vi "校准测试.vi"(8 "error in (no error)":errorcluster, 9 "out":i32=1, 11 "in":i32=2) -> (0 "error out":errorcluster)   [LabVIEW 2015]
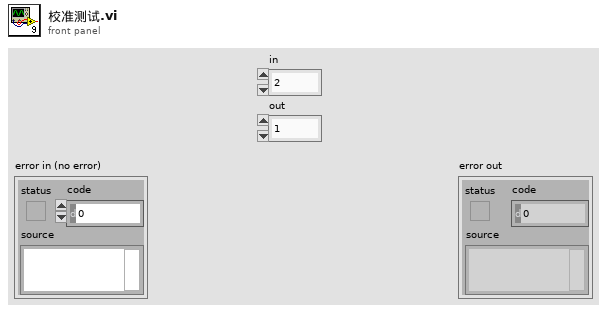
[diagram p1: front panel]
types:
  T1 = typedef "直通基准state.ctl" = enum16{"Idle", "开始消息", "切换开关", "网分测量", "数据库操作", "结束消息"}
  T2 = cluster{"Freq":dbl[], "S11":dbl[], "S12":dbl[], "S21":dbl[], "S22":dbl[]}
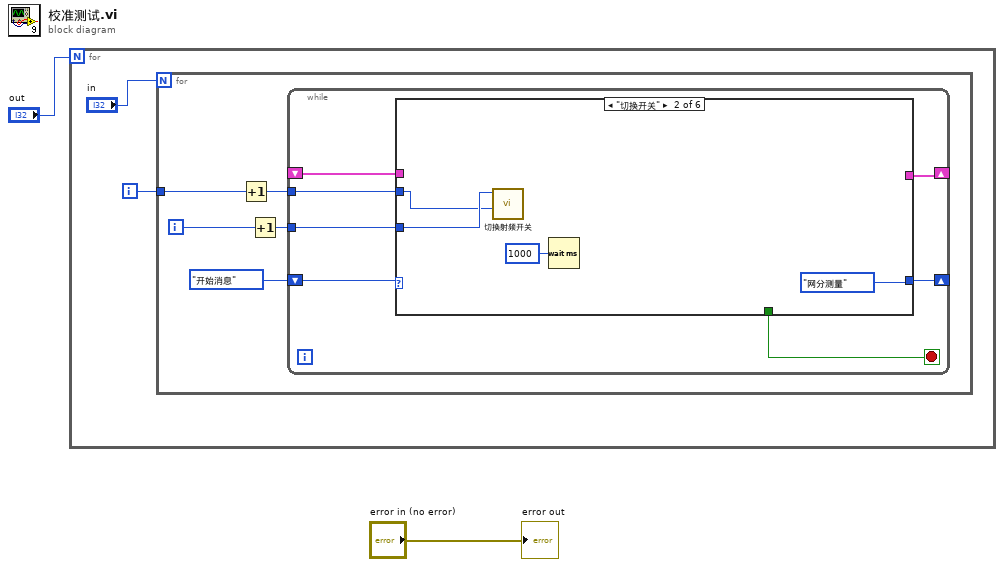
[diagram p0: block diagram]
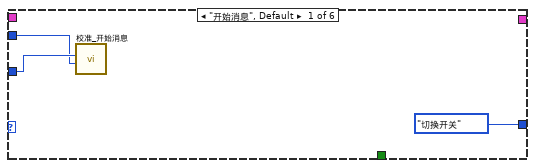
[diagram p2: hidden frame]
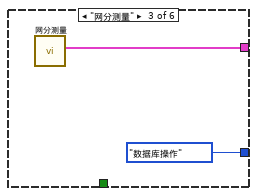
[diagram p3: hidden frame]
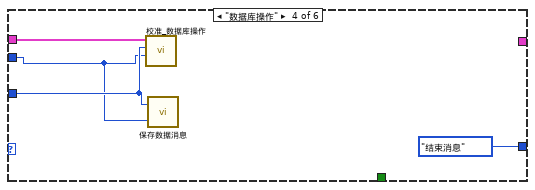
[diagram p4: hidden frame]
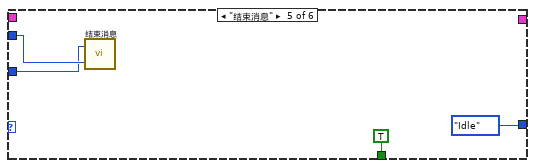
[diagram p5: hidden frame]
diagram:
  n1 = for {
    N: "out" -> [_]
    i -> [w4]
    n2 = for {
      N: "in" -> [_]
      tunnel: w4 -> [w9]
      i -> [w8]
      n3 = Increment(x=w9) -> (x+1=w7:i32)
      n4 = Increment(x=w8) -> (x+1=w6:i32)
      n5 = while {
        tunnel: w7 -> [w16]
        tunnel: w6 -> [w15]
        shift-right: [w13] -> _
        shift-left: 直通基准state."开始消息" ("直通基准State") -> [w14]
        shift-right: [w11] -> _
        shift-left: _ -> [w10]
        stop <- w12 stop-if-true
        n6 = case shown="\"切换开关\"" w14 {
          tunnel: w16 -> [w17 w20 _ w26 w31 _]
          tunnel: w15 -> [w18 w21 _ w27 w30 _]
          tunnel: [直通基准state."切换开关" ("直通基准State") 直通基准state."网分测量" ("直通基准State") 直通基准state."数据库操作" ("直通基准State") 直通基准state."结束消息" ("直通基准State") 直通基准state."Idle" ("直通基准State") _] -> w13
          tunnel: [_ _ _ _ TRUE _] -> w12
          tunnel: [_ _ w25 _ _ _] -> w11
          tunnel: w10 -> [_ _ _ w29 _ _]
          frame "开始消息", Default {
            n7 = call "校准_开始消息.vi"("COM"=w17, "A"=w18) -> ()  [unwired: 10 in]
          }
          frame "切换开关" {
            n8 = call "切换射频开关.vi"("COM"=w20, "A"=w21) -> ()  [unwired: 7 in, 3 out]
            n9 = Wait (ms)(milliseconds to wait=u32 1000) -> ()  [unwired: 1 out]
          }
          frame "网分测量" {
            n10 = call "网分测量.vi"() -> ("Freq&S"=w25:T2)  [unwired: 11 in]
          }
          frame "数据库操作" {
            n11 = call "校准_数据库操作.vi"("出口"=w26, "进口"=w27, "Freq&S"=w29) -> ()  [unwired: 8 in, 1 out]
            n12 = call "保存数据消息.vi"("COM"=w26, "A"=w27) -> ()  [unwired: 1 in]
          }
          frame "结束消息" {
            n13 = call "结束消息.vi"("COM"=w31, "A"=w30) -> ()  [unwired: 1 in]
          }
          frame "Idle" {
          }
        }
      }
    }
  }
  "error out" <- "error in (no error)"
